vi "Find out what this is.vi"   [LabVIEW 2021]
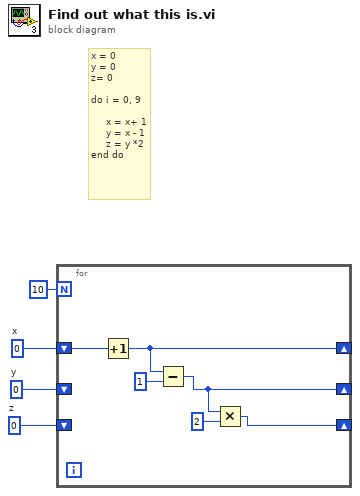
[diagram p0: block diagram]
diagram:
  w1 = 0  # z
  w2 = 0  # y
  w3 = 0  # x
  # "x = 0 \ny = 0\nz= 0\n\ndo i = 0, 9\n\n     x = x+ 1\n     y = x - 1\n     z = y *2\nend do"
  n1 = for {
    N: 10 -> [_]
    shift-right: [w9] -> _
    shift-left: w3 -> [w10]
    shift-right: [w7] -> _
    shift-left: w2 -> [_]
    shift-right: [w5] -> _
    shift-left: w1 -> [_]
    n2 = Increment(x=w10) -> (x+1=w9:i32)
    n3 = Subtract(x=w9, y=1) -> (x-y=w7:i32)
    n4 = Multiply(x=w7, y=2) -> (x*y=w5:i32)
  }
